vi "[FPGA] TIntegralR Multichannel.vi"(0 "x{k}":sgl, 1 "reset":bool, 5 "x^2?":bool, 7 "zero cross direction":enum8{"either", "minus-plus", "plus-minus"}(ring), 9 "Debounce (iterations)":i32=1, 11 "dt (s)":sgl, 13 "Channel #":u32) -> (4 "TIntegralR(x{k})":sgl, 10 "dT [s]":sgl)   [LabVIEW 2015]
uses:
  Floating Point/Polymorphic subVIs/Multiply 00.vi
  <vilib>/rvi/DataTransferAndStorage/Container/Common/niFpgaContainerGetUniqueNameForEmu.vi
  <vilib>/rvi/DataTransferAndStorage/Container/Common/niFpgaContainerSetEmuInfo.vi
  <vilib>/rvi/eio/common/nirviEmuReportErrorAndStop.vi
  <vilib>/rvi/DataTransferAndStorage/Container/Common/niFpgaContainerExecOnDevCompGetState.vi
  <vilib>/rvi/Emulation/niFpgaEmulationIsFPGAContextNoSignature.vi
  <vilib>/rvi/Emulation/niFpgaProcessEmulError.vi
  <vilib>/rvi/Emulation/niFpgaSctlEmulationGetInTimedLoop.vi
  <vilib>/rvi/errors/nirviReportUnexpectedCaseInternalError (U32).vi
  <vilib>/rvi/Memory/Memory_Emulation/niFpgaMemoryEmulationCacheClearOnFirstRun.vi
  <vilib>/rvi/Memory/Memory_Emulation/nirvimemoryEmulationManagerCache_MakeExclusive.vi
  <vilib>/rvi/Memory/Memory_Emulation/niFpgaMemoryEmulationValidateCache.vi
  <vilib>/rvi/Memory/Memory_Emulation/nirvimemoryEmulationManagerCache_InsertValue.vi
  <vilib>/Utility/error.llb/Clear Errors.vi
  <vilib>/rvi/Memory/Memory_Emulation/nirvimemoryEmulationManagerCache_ReleaseExclusive.vi
  <vilib>/rvi/Memory/Memory_Emulation/nirvimemoryEmulationManagerCache_GetValue.vi
  <vilib>/rvi/Memory/Memory_Emulation/nirvimemoryEmulationManagerCache_SetValue.vi
  <vilib>/rvi/Emulation/niFpgaSctlEmulationResourceMgr.vi
  Floating Point/Polymorphic subVIs/Add 00.vi
  <vilib>/rvi/LocalResourceManager/LocalResourceManager.xnode
  <vilib>/rvi/DataTransferAndStorage/Container/XNode/niFpgaContainer.xnode
  <vilib>/rvi/Memory/Memory_Emulation/niFpgaMemoryEmulationRefIn.vi
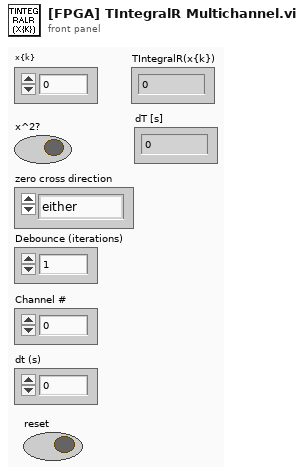
[diagram p1: front panel]
types:
  T1 = cluster{"yi{k-1} ":sgl, "xi{k-1}":sgl, "yo":sgl, "dT [s]":sgl, "To [Ticks]":u32}
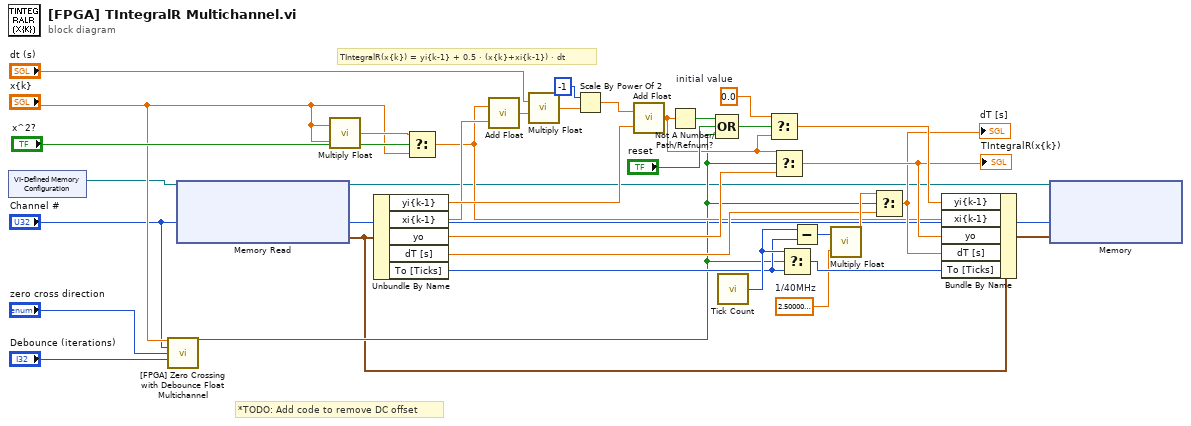
[diagram p0: block diagram]
diagram:
  w19 = sgl 2.5e-08  # 1/40MHz
  w31 = sgl 0.0  # initial value
  # "*TODO: Add code to remove DC offset"
  # "TIntegralR(x{k}) = yi{k-1} + 0.5 · (x{k}+xi{k-1}) · dt"
  n1 = xnode ("VI-Defined Memory Configuration")() -> ("Memory Out"=w5:refnum<k21>)
  n2 = call "[FPGA] Zero Crossing with Debounce Float Multichannel.vi"("input"="x{k}", "Channel #"="Channel #", "direction"="zero cross direction", "Debounce (iterations)"="Debounce (iterations)") -> ("crossing"=w7:bool)  [unwired: 11 in]
  n3 = xnode "Memory Read"("Address"="Channel #", "Memory In"=w5) -> ("Data"=w4:T1, "Memory Out"=w3:refnum<k21>)
  n4 = call-poly "Multiply Float.vi"("y"="x{k}", "x"="x{k}") -> ("x*y"=w10:sgl)
  n5 = Unbundle By Name(w4) -> ("yi{k-1}"=w34:sgl, "xi{k-1}"=w33:sgl, "yo"=w25:sgl, "dT [s]"=w16:sgl, "To [Ticks]"=w20:u32)
  n6 = Select(t=w10, s="x^2?", f="x{k}") -> (s? t:f=w8:sgl)
  n7 = call-poly "Add Float.vi"("y"=w33, "x"=w8) -> ("x+y"=w14:sgl)
  n8 = call-poly "Multiply Float.vi"("y"=w14, "x"="dt (s)") -> ("x*y"=w13:sgl)
  n9 = Scale By Power Of 2(n=i8 -1, x=w13) -> (x*2^n=w11:sgl)
  n10 = call-poly "Add Float.vi"("y"=w34, "x"=w11) -> ("x+y"=w26:sgl)
  n11 = Not A Number/Path/Refnum?(number/path/refnum=w26) -> (NaN/Path/Refnum?=w32:bool)
  n12 = Compound Arithmetic op=OR(w32, "reset", w7) -> (w24:bool)
  n13 = call "Tick Count"() -> ("Tick Count(Ticks)"=w21:u32)
  n14 = Select(t=w31, s=w24, f=w26) -> (s? t:f=w29:sgl)
  n15 = Select(t=w26, s=w7, f=w25) -> (s? t:f=w22:sgl)
  "TIntegralR(x{k})" <- w22
  n16 = Select(t=w21, s=w7, f=w20) -> (s? t:f=w23:u32)
  n17 = Subtract(x=w21, y=w20) -> (x-y=w18:u32)
  n18 = call-poly "Multiply Float.vi"("y"=w19, "x"=w18) -> ("x*y"=w17:sgl)
  n19 = Select(t=w17, s=w7, f=w16) -> (s? t:f=w15:sgl)
  "dT [s]" <- w15
  n20 = Bundle By Name(cluster=w4, "yi{k-1}"=w29, "xi{k-1}"=w8, "yo"=w22, "dT [s]"=w15, "To [Ticks]"=w23) -> (w1:T1)
  n21 = xnode "Memory"("Address"="Channel #", "Data"=w1, "Memory In"=w3) -> ()  [unwired: 1 out]
